vi "Launch.vi"(4 "Sub Panel":refnum<vi>, 6 "Launch Timeout [ms]":i32=-1, 8 "error in (no error)":errorcluster) -> (0 "error out":errorcluster, 1 "Title":string, 2 "Launch Time":timestamp, 3 "Actor API out":refnum<class "Actor API.lvclass">)   [LabVIEW 2015, in "Info View.lvclass"]
doc: "<b>Response</b> channel is used by this actor to return infomation back to the parent. Typically this input is the Request channel of the parent actor."
uses:
  Info View.lvclass
  Re-use Libraries/Minimal Actor Framework/Actors/Base Actor/API/Actor API.lvclass
  Re-use Libraries/Minimal Actor Framework/Messaging/Messenger/Messenger.lvclass
  Re-use Libraries/Minimal Actor Framework/Actors/Base Actor/Actor/Front Panel State.ctl
  Re-use Libraries/Minimal Actor Framework/Actors/Base Actor/Actor/Actor.lvclass
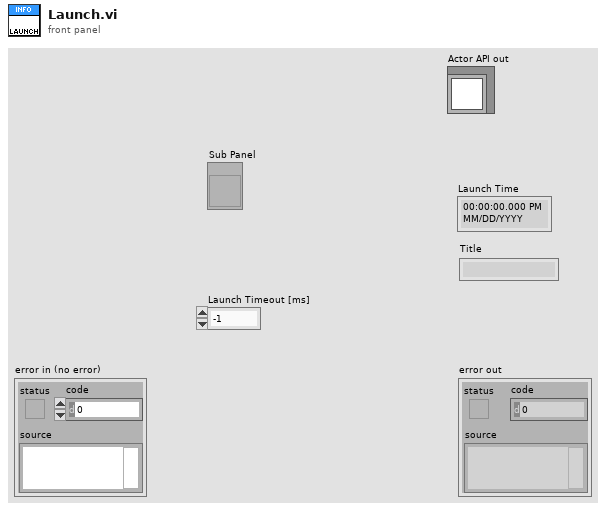
[diagram p1: front panel]
types:
  T1 = typedef "Actor.lvclass/Front Panel State.ctl" = enum32{"Invalid", "Standard", "Closed", "Hidden", "Minimized", "Maximized"}
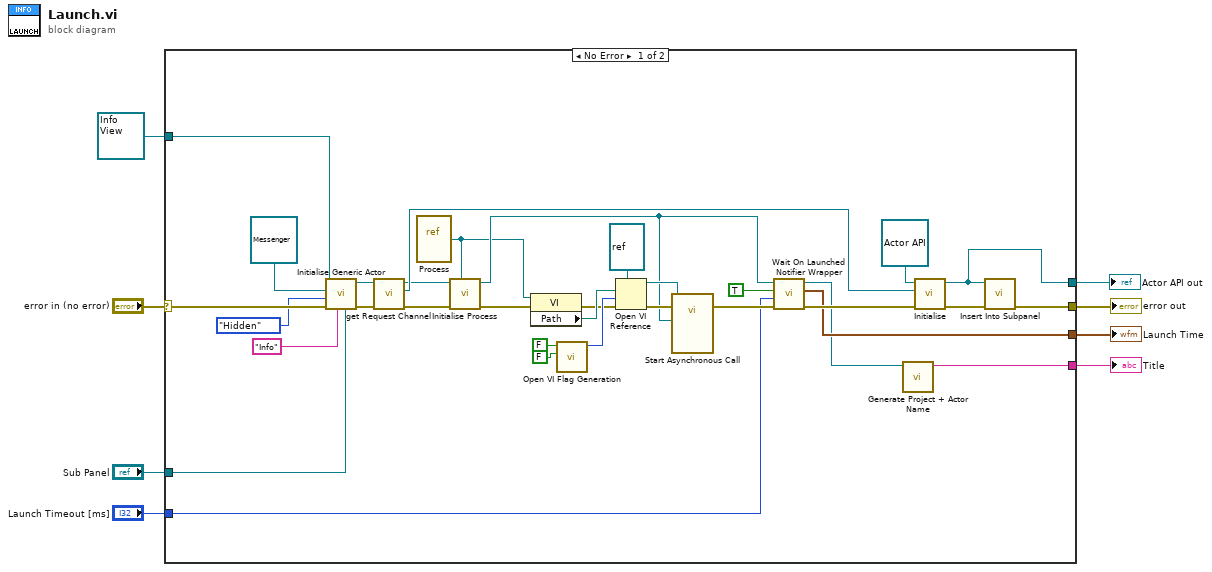
[diagram p0: block diagram]
diagram:
  n1 = case shown="No Error" "error in (no error)" {
    selector: "error in (no error)" -> [w32 w41]
    tunnel: [w21 w41] -> w8
    tunnel: [w10 _] -> w1
    tunnel: refnum<class "Info View.lvclass"> refnum ("Worker Test 1.lvclass") -> [w9 _]
    tunnel: "Sub Panel" -> [w31 _]
    tunnel: "Launch Timeout [ms]" -> [w28 _]
    tunnel: [w27 _] -> w3
    tunnel: [w17 _] -> w2
    frame No Error {
      n2 = call-dynamic "Initialise Generic Actor.vi"("Sub Panel"=w31, "Name"="Info", "Front Panel State"=Front_Panel_State."Hidden", "Response Channel"=refnum<class "Messenger.lvclass"> refnum, "Actor in"=w9) -> ("Actor out"=w33:refnum<class "Info View.lvclass">)  [unwired: 5 in, 1 out]
      n3 = call "get Request Channel.vi"("error in (no error)"=w32, "Actor in"=w33) -> ("error out"=w15:errorcluster, "Request Channel"=w34:refnum<class "Messenger.lvclass">, "Actor out"=w14:refnum<class "Info View.lvclass">)  [unwired: 7 in]
      n4 = vi-ref "Process.vi"() -> (w11:refnum<vi>)
      n5 = call-dynamic "Initialise Process.vi"("Process"=w11, "error in (no error)"=w15, "Actor in"=w14) -> ("error out"=w12:errorcluster, "Actor out"=w13:refnum<class "Info View.lvclass">)  [unwired: 7 in]
      n6 = property class="VI"(reference=w11, error in=w12) -> (error out=w19:errorcluster, "Path"=w20:path)  [unwired: 1 out]
      n7 = call "Open VI Flag Generation.vi"("Call And Collect (F)"=FALSE, "Re-entrant (F)"=FALSE) -> ("Flags"=w40:i32)  [unwired: 9 in]
      n8 = Open VI Reference(type specifier VI Refnum (for type only)=refnum<vi> refnum, vi path=w20, options=w40, error in (no error)=w19) -> (vi reference=w36:refnum<vi>, error out=w35:errorcluster)  [unwired: 2 in]
      n9 = call-by-ref "Start Asynchronous Call"(reference=w36, error in=w35, "Worker Test 1.lvclass"=w13) -> (error out=w30:errorcluster)  [unwired: 11 in, 1 out]
      n10 = call-dynamic "Wait On Launched Notifier Wrapper.vi"("error in (no error)"=w30, "Launch Timeout [ms]"=w28, "Wait For Launch Completed"=TRUE ("Wait For Launch Completed (F)"), "Actor in"=w13) -> ("error out"=w29:errorcluster, "Launch Time"=w27:timestamp, "Actor out"=w18:refnum<class "Info View.lvclass">)  [unwired: 5 in]
      n11 = call "Generate Project + Actor Name.vi"("Actor in"=w18) -> ("concatenated string"=w17:string)  [unwired: 10 in]
      n12 = call "Initialise.vi"("error in (no error)"=w29, "Request Channel"=w34, "Actor API in"=refnum<class "Actor API.lvclass"> refnum ("Actor API.lvclass")) -> ("error out"=w22:errorcluster, "Actor API out"=w10:refnum<class "Actor API.lvclass">)  [unwired: 7 in]
      n13 = call-dynamic "Insert Into Subpanel.vi"("error in (no error)"=w22, "Actor API in"=w10) -> ("error out"=w21:errorcluster)  [unwired: 9 in]
    }
    frame Error {
    }
  }
  "error out" <- w8
  "Launch Time" <- w3
  "Title" <- w2
  "Actor API out" <- w1
